vi "Verificar advertencias.vi"(8 "error in":errorcluster, 11 "VISA COM IN":refnum<visa-resource-name>) -> (0 "error out":errorcluster, 3 "VISA COM OUT":refnum<visa-resource-name>)   [LabVIEW 2011]
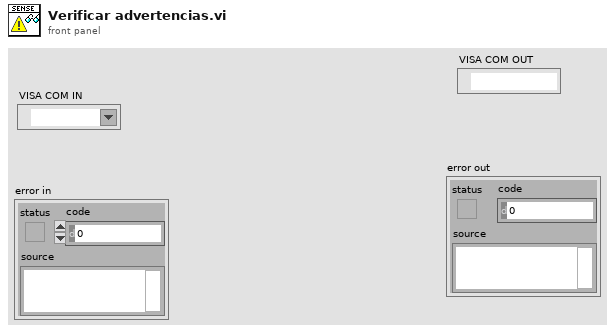
[diagram p1: front panel]
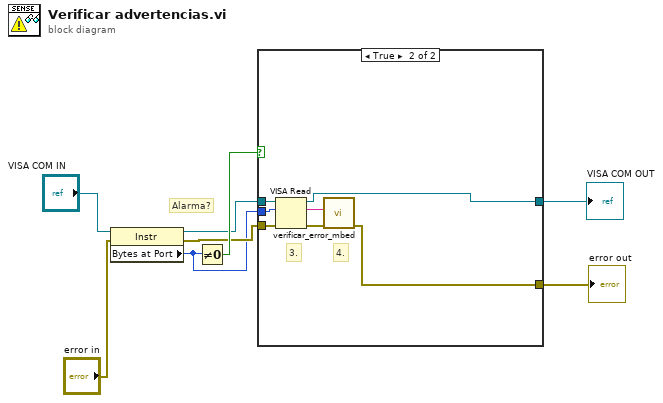
[diagram p0: block diagram]
diagram:
  # "Alarma?"
  n1 = property class="Instr"(reference="VISA COM IN", error in="error in") -> (reference out=w6:refnum<visa-resource-name>, error out=w5:errorcluster, "Bytes at Port"=w4:u32)
  n2 = Not Equal To 0?(x=w4) -> (x != 0?=w8:bool)
  n3 = case shown="True" w8 {
    tunnel: w6 -> [w10 w15]
    tunnel: w5 -> [w9 w14]
    tunnel: w4 -> [_ w13]
    tunnel: [w10 w12] -> w3
    tunnel: [w9 w11] -> w2
    frame False {
    }
    frame True {
      # "4."
      # "3."
      n4 = VISA Read(VISA resource name=w15, byte count=w13, error in (no error)=w14) -> (VISA resource name out=w12:refnum<visa-resource-name>, read buffer=w16:string, error out=w17:errorcluster)  [unwired: 1 out]
      n5 = call "verificar_error_mbed.vi"("error in (no error)"=w17, "desde_mbed"=w16) -> ("error out"=w11:errorcluster)  [unwired: 8 in, 1 out]
    }
  }
  "VISA COM OUT" <- w3
  "error out" <- w2
